vi "Field Draw Future Robot.vi"(4 "Lado":enum16{"Esquerdo", "Direito"}(ring) caption="Enum", 6 "Draw Targets?":T1, 7 "Robot 2":refnum<class "Robot.lvclass">, 8 "Scale mm/pixel":dbl, 9 "Offset":T2, 11 "picture in":picture) -> (2 "picture out":picture)   [LabVIEW 2023]
uses:
  <vilib>/Utility/miscctls.llb/LVBoundsTypeDef.ctl
  DrawTargets.ctl
  Robot_class/Robot.lvclass
  Object_class/Object.lvclass/Object.ctl
  Object_class/Read x.vi
  Object_class/Read y.vi
  Object_class/Read pos_est_x.vi
  Object_class/Read pos_est_y.vi
  <vilib>/Analysis/NI_AALPro.lvlib
  <vilib>/Analysis/coordinate.llb/2D Cartesian Coordinate Rotation (Scalar).vi
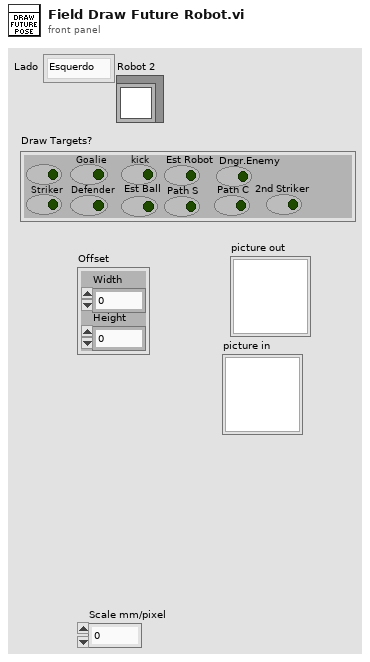
[diagram p1: front panel]
types:
  T1 = typedef "DrawTargets.ctl" = cluster{"Attacker":bool, "Striker":bool, "Goalie":bool, "Defender":bool, "kick":bool, "Est Ball":bool, "Est Robot":bool, "Path S":bool, "Path C":bool, "Dngr.Enemy":bool, "2nd Striker":bool}
  T2 = typedef "LVBoundsTypeDef.ctl" = cluster{"Width":u32, "Height":u32}
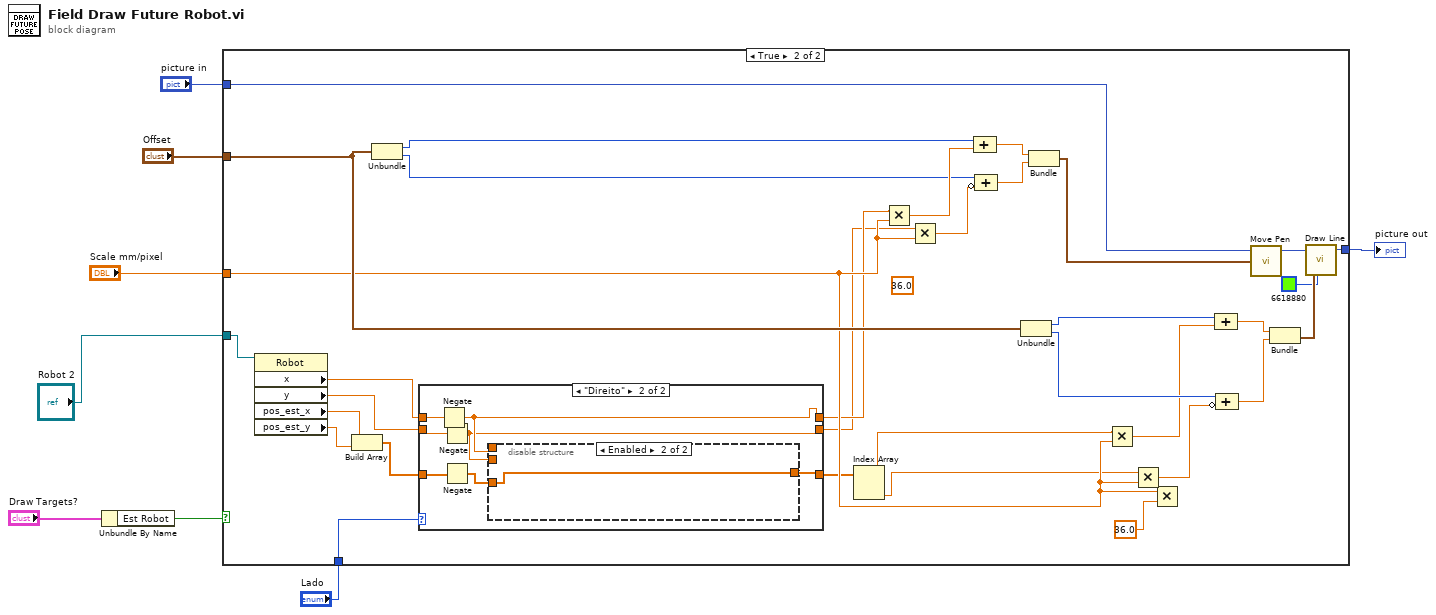
[diagram p0: block diagram]
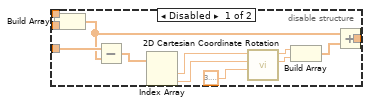
[diagram p4: hidden frame]
diagram:
  n1 = Unbundle By Name("Draw Targets?") -> ("Est Robot"=w3:bool)
  n2 = case shown="True" w3 {
    tunnel: [w9 w36] -> w8
    tunnel: "Offset" -> [_ w30]
    tunnel: "Scale mm/pixel" -> [_ w27]
    tunnel: "picture in" -> [w9 w21]
    tunnel: "Lado" -> [_ w19]
    tunnel: "Robot 2" -> [_ w15]
    frame False {
    }
    frame True {
      (unwired) sgl 36.0 ("radius")
      n3 = property class="Robot"(reference=w15) -> ("x"=w10:dbl, "y"=w11:dbl, "pos_est_x"=w14:dbl, "pos_est_y"=w13:dbl)  [unwired: 1 in, 2 out]
      n4 = Build Array(w14, w13) -> (w12:dbl[])
      n5 = Unbundle(w30) -> ("Width"=w42:u32, "Height"=w39:u32)
      n6 = case shown="\"Direito\"" w19 {
        tunnel: [w45 w49] -> w18
        tunnel: w10 -> [w45 w52]
        tunnel: [w44 w48] -> w17
        tunnel: w11 -> [w44 w51]
        tunnel: [w43 w46] -> w16
        tunnel: w12 -> [w43 w50]
        frame "Esquerdo", Default {
        }
        frame "Direito" {
          n7 = Negate(x=w52) -> (-x=w49:dbl)
          n8 = Negate(x=w51) -> (-x=w48:dbl)
          n9 = Negate(x=w50) -> (-x=w47:dbl[])
          n10 = disable-structure shown="Enabled" {
            disable-tunnel: w49 -> [w59 _]
            disable-tunnel: w48 -> [w58 _]
            disable-tunnel: w47 -> [w57 w65]
            disable-tunnel: [w55 w65] -> w46
            frame Disabled {
              n11 = Build Array(w59, w58) -> (w53:dbl[])
              n12 = Subtract(x=w57, y=w53) -> (x-y=w56:dbl[])
              n13 = Index Array(array=w56) -> (element #1=w64:dbl, element #2=w63:dbl)  [unwired: 2 in]
              n14 = call-poly <vilib>:"2D Cartesian Coordinate Rotation.vi"("theta"=3.141592653589793, "y"=w63, "x"=w64) -> ("y out"=w61:dbl, "x out"=w62:dbl)  [unwired: 6 in, 1 out]
              n15 = Build Array(w62, w61) -> (w54:dbl[])
              n16 = Add(x=w53, y=w54) -> (x+y=w55:dbl[])
            }
            frame Enabled {
            }
          }
        }
      }
      n17 = Index Array(array=w16) -> (element #1=w24:dbl, element #2=w23:dbl)  [unwired: 2 in]
      n18 = Multiply(x=w18, y=w27) -> (x*y=w41:dbl)
      n19 = Multiply(x=w17, y=w27) -> (x*y=w38:dbl)
      n20 = Compound Arithmetic op=ADD(w42, w41) -> (w40:dbl)
      n21 = Compound Arithmetic op=ADD(w39, invert w38) -> (w37:dbl)
      n22 = Unbundle(w30) -> ("Width"=w34:u32, "Height"=w32:u32)
      n23 = Bundle(w40, w37) -> (w20:cluster{dbl, dbl})  [unwired: 1 in]
      n24 = Multiply(x=w24, y=w27) -> (x*y=w26:dbl)
      n25 = Multiply(x=w23, y=w27) -> (x*y=w25:dbl)
      n26 = Multiply(x=w27, y=sgl 36.0 ("radius")) -> ()  [unwired: 1 out]
      n27 = Compound Arithmetic op=ADD(w34, w26) -> (w33:dbl)
      n28 = Compound Arithmetic op=ADD(w32, invert w25) -> (w31:dbl)
      n29 = call <vilib>:"Move Pen.vi"("new position"=w20, "picture"=w21) -> ("new picture"=w35:picture)  [unwired: 3 in]
      n30 = Bundle(w33, w31) -> (w29:cluster{dbl, dbl})  [unwired: 1 in]
      n31 = call <vilib>:"Draw Line.vi"("picture"=w35, "end point"=w29, "color(black)"=u32 6618880) -> ("new picture"=w36:picture)  [unwired: 6 in]
    }
  }
  "picture out" <- w8
